vi "ELVIS III v1.0 RPC Heart Beat Thread.vi"   [LabVIEW 2021]
uses:
  <vilib>/myRIO/Common/Instrument Driver Framework/ELVIS III v1.0/Resource Manager/typedefs/ELVIS III v1.0 RIO Session Map Action.ctl
types:
  T1 = typedef "ELVIS III v1.0 RIO Session Map Action.ctl" = enum16{"Add Session", "Remove Session", "Get Active Sessions", "Get Owning Sessions"}
  T2 = cluster{"Session":u32, "Channel Names":string[]}[]
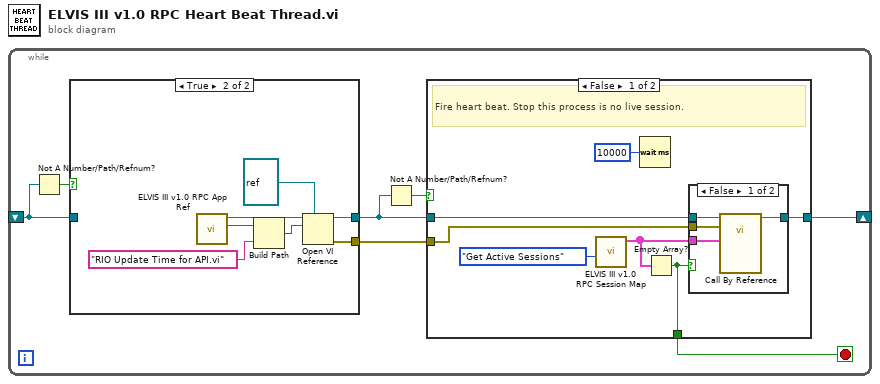
[diagram p0: block diagram]
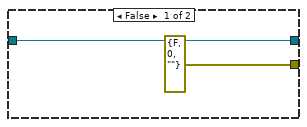
[diagram p2: hidden frame]
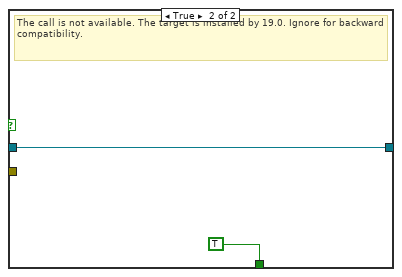
[diagram p4: hidden frame]
diagram:
  n1 = while {
    shift-right: [w5] -> _
    shift-left: _ -> [w3]
    stop <- w1 stop-if-true
    n2 = Not A Number/Path/Refnum?(number/path/refnum=w3) -> (NaN/Path/Refnum?=w4:bool)
    n3 = case shown="True" w4 {
      tunnel: [w9 w16] -> w6
      tunnel: w3 -> [w9 _]
      tunnel: [errorcluster {"status"=FALSE, "code"=0, "source"=""} ("error out") w15] -> w2
      frame False {
      }
      frame True {
        n4 = call <vilib>:"ELVIS III v1.0 RPC App Ref.vi"() -> ("Lib Path"=w11:path, "RPC Reference"=w13:refnum<vi>)  [unwired: 10 in]
        n5 = Build Path(base path=w11, name or relative path="RIO Update Time for API.vi") -> (appended path=w10:path)
        n6 = Open VI Reference(type specifier VI Refnum (for type only)=refnum<vi> refnum, application reference (local)=w13, vi path=w10) -> (vi reference=w16:refnum<vi>, error out=w15:errorcluster)  [unwired: 3 in]
      }
    }
    n7 = Not A Number/Path/Refnum?(number/path/refnum=w6) -> (NaN/Path/Refnum?=w7:bool)
    n8 = case shown="False" w7 {
      tunnel: w6 -> [w23 w30]
      tunnel: [w22 w30] -> w5
      tunnel: w2 -> [w21 _]
      tunnel: [w17 TRUE ("Stop")] -> w1
      frame False {
        # "Fire heart beat. Stop this process is no live session."
        n9 = call <vilib>:"ELVIS III v1.0 RPC Session Map.vi"("Action"=ELVIS_III_v1.0_RIO_Session_Map_Action."Get Active Sessions" ("Session Map Action")) -> ("Session Infos"=w19:T2)  [unwired: 9 in, 1 out]
        n10 = Wait (ms)(milliseconds to wait=u32 10000) -> ()  [unwired: 1 out]
        n11 = Empty Array?(array=w19) -> (empty?=w17:bool)
        n12 = case shown="False" w17 {
          tunnel: w23 -> [w27 w28]
          tunnel: [w26 w28] -> w22
          tunnel: w21 -> [w25 _]
          tunnel: w19 -> [w24 _]
          frame False {
            n13 = call-by-ref "?"(reference=w27, error in=w25, "Session Infos"=w24) -> (reference out=w26:refnum<vi>)  [unwired: 9 in, 3 out]
          }
          frame True {
          }
        }
      }
      frame True {
        # "The call is not available. The target is installed by 19.0. Ignore for backward compatibility."
      }
    }
  }
